vi "PCF8591_AI.vi"(8 "error in (no error)":errorcluster, 11 "Channel":enum16{"CH0", "CH1", "CH2", "CH3"}(ring)) -> (0 "error out":errorcluster, 3 "Data":i32)   [LabVIEW 2014, in "QwaveSys Raspberry Pi Library.lvlib"]
uses:
  QwaveSys Raspberry Pi Library.lvlib
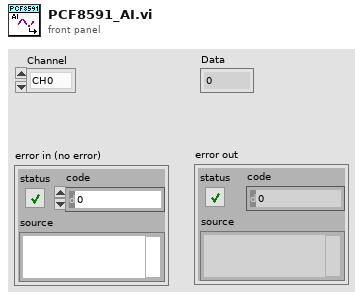
[diagram p1: front panel]
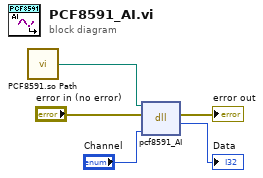
[diagram p0: block diagram]
diagram:
  n1 = call "PCF8591.so Path.vi"() -> ("PCF8591.so Path"=w3:path)  [unwired: 5 in]
  n2 = dll-call lib="pcf8591.so" fn="pcf8591_AI"(path in=w3, error in="error in (no error)", "pin"="Channel") -> (error out=→"error out":errorcluster, "return type"=→"Data":i32)  [unwired: 2 in, 1 out]
